vi "DC Voltmeter.vi"() -> ()   [LabVIEW 2017]
panel:
  out "error out":errorcluster
  in  "stop":bool
  out "Voltage":dbl format="%.4g"
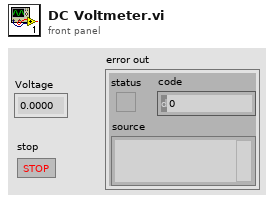
[diagram p1: front panel]
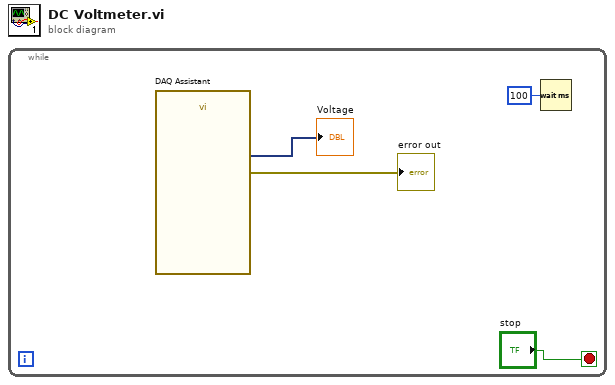
[diagram p0: block diagram]
diagram:
  n1 = while {
    stop <- "stop" stop-if-true
    n2 = call "DAQ Assistant"() -> ("data"=→"Voltage":dynamicdata, "error out"=→"error out":errorcluster)  [unwired: 17 in, 1 out]
    n3 = Wait (ms)(milliseconds to wait=u32 100) -> ()  [unwired: 1 out]
  }
